vi "Read Rank.vi"(8 "error in":errorcluster, 11 "SG Path Group in":refnum<class "SG Path Group.lvclass">) -> (0 "error out":errorcluster, 2 "Rank":dbl, 3 "SG Path Group out":refnum<class "SG Path Group.lvclass">)   [LabVIEW 2023, in "RFFixtureCharact.RMM.lvlib" / "SG Path Group.lvclass"]
uses:
  SG Path Group.lvclass
  SG Path Group.lvclass/SG Path Group.ctl
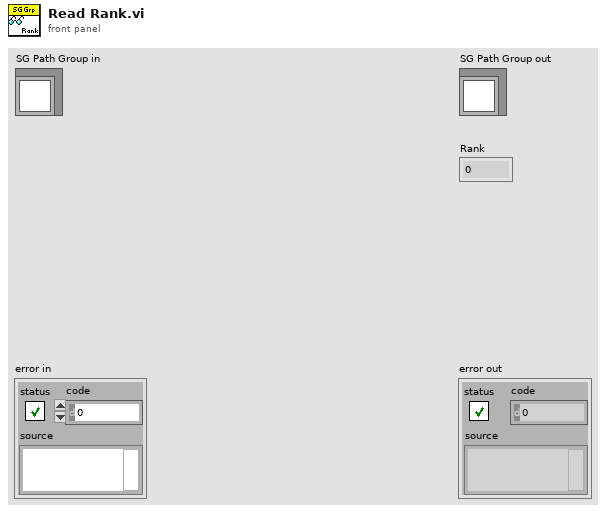
[diagram p1: front panel]
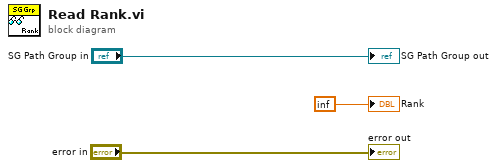
[diagram p0: block diagram]
diagram:
  "error out" <- "error in"
  "SG Path Group out" <- "SG Path Group in"
  "Rank" <- inf
